vi "Draw Gates On XY Chart.vi"(7 "Micropulse No.":i32, 8 "error in (no error)":errorcluster, 9 "Echo Range":dbl, 10 "XYGraph in":refnum<vi>, 11 "Test No.":u32) -> (0 "error out":errorcluster)   [LabVIEW 2026, in "MicroPulse_Driver.lvlib"]
uses:
  <instrlib>/MicroPulse/MicroPulse_Driver.lvlib
panel:
  out "Picture out":picture
  in  "Picture in":picture
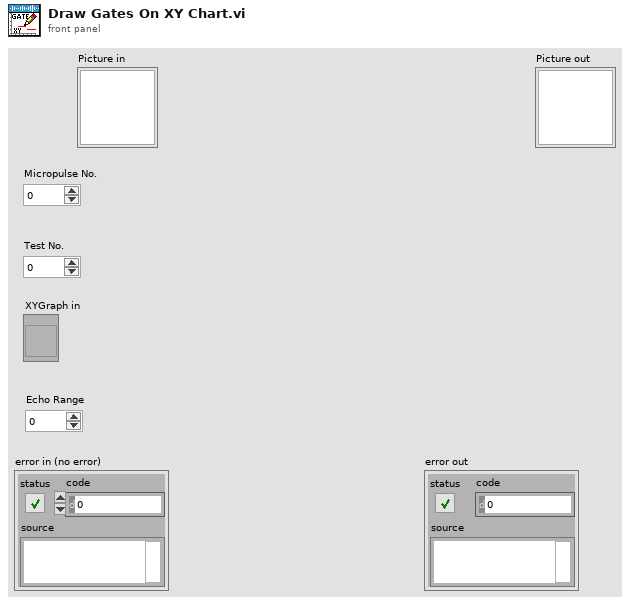
[diagram p1: front panel]
types:
  T1 = cluster{"Start (us)":dbl, "Length (us)":dbl, "Threshold":u16, "Name":string, "Enabled?":bool, "Colour":u32}
  T2 = cluster{"Lable":string, "Visible":bool, "Width":u16, "Colour":u32, "Line":enum32{"Solid", "Dash", "Dot", "DashDot", "DashDotDot"}}
  T3 = typedef "MicroPulse_Driver.lvlib/MP - Registry Gates.ctl" = cluster{"Display Gate":T4, "ETM Mode":T5, "Echo Gate":T6, "Insp Gates":T7[]}
  T4 = typedef "MicroPulse_Driver.lvlib/MP - display gate.ctl" = cluster{"Start":dbl, "Length":dbl}
  T5 = typedef "MicroPulse_Driver.lvlib/MP - echo gate mode.ctl" = enum16{"Echo Trigger OFF", "Echo Gate Display Mode", "Echo Trigger ON", "Multi Gate or FMC Mode", "Reserved", "PA - Echo Trigger ON"}
  T6 = typedef "MicroPulse_Driver.lvlib/MP - echo gate parameters.ctl" = cluster{"Start (us)":dbl, "Length (us)":dbl, "Threshold":u16, "Colour":u32}
  T7 = typedef "MicroPulse_Driver.lvlib/MP - multigate inspection gate parameters.ctl" = cluster{"Start (us)":dbl, "Length (us)":dbl, "Threshold":u16, "Enabled?":bool, "Max # Peaks":u16, "Hysteresis":T8, "Mode":T9, "Inverted?":bool, "Colour ":u32}
  T8 = typedef "MicroPulse_Driver.lvlib/MP - hysteresis level.ctl" = enum16{"None", "3dB", "6dB", "9dB", "12dB"}
  T9 = typedef "MicroPulse_Driver.lvlib/MP - multigate mode.ctl" = enum16{"1st Peak in Gate", "Largest Peak In Gate", "All Peaks In Gate", "1st Threshold Crossing"}
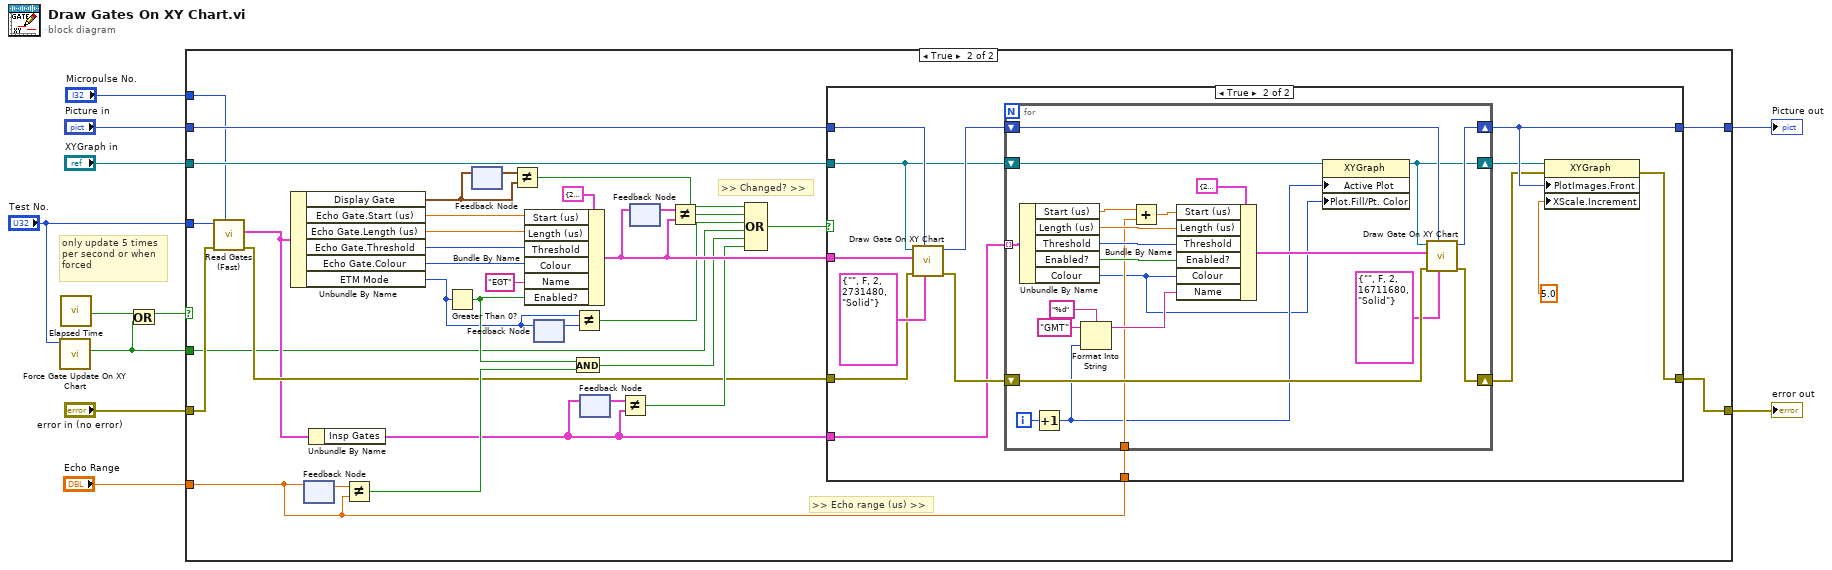
[diagram p0: block diagram]
diagram:
  # "only update 5 times\nper second or when\nforced"
  n1 = call <instrlib>:"Force Gate Update On XY Chart.vi"("Test No."="Test No.") -> ("Update gate display?"=w1:bool)  [unwired: 8 in, 2 out]
  n2 = call "Elapsed Time"() -> ("Time has Elapsed"=w4:bool)  [unwired: 12 in, 7 out]
  n3 = Or(x=w4, y=w1) -> (x .or. y?=w3:bool)
  n4 = case shown="True" w3 {
    tunnel: [w13 w47] -> w11
    tunnel: [w12 w46] -> w10
    tunnel: "Picture in" -> [w13 w45]
    tunnel: "XYGraph in" -> [_ w44]
    tunnel: "Test No." -> [_ w20]
    tunnel: "error in (no error)" -> [w12 w32]
    tunnel: "Micropulse No." -> [_ w30]
    tunnel: "Echo Range" -> [_ w15]
    tunnel: w1 -> [_ w14]
    frame False {
    }
    frame True {
      # ">> Echo range (us) >>"
      # ">> Changed? >>"
      n5 = call <instrlib>:"Read Gates (Fast).vi"("Micropulse # In"=w30, "error in (no error)"=w32, "Test No."=w20) -> ("error out"=w31:errorcluster, "Gates"=w29:T3)  [unwired: 5 in, 2 out]
      n6 = Unbundle By Name(w29) -> ("Display Gate"=w26:T4, "Echo Gate.Start (us)"=w43:dbl, "Echo Gate.Length (us)"=w42:dbl, "Echo Gate.Threshold"=w41:u16, "Echo Gate.Colour"=w16:u32, "ETM Mode"=w17:T5)
      n7 = feedback #1() -> (w35:dbl)  [unwired: 1 in]
      n8 = feedback-in #1(w15) -> ()
      n9 = Unbundle By Name(w29) -> ("Insp Gates"=w28:T7[])
      n10 = Not Equal?(x=w35, y=w15) -> (x != y?=w34:bool)
      n11 = Greater Than 0?(x=w17) -> (x > 0?=w18:bool)
      n12 = feedback #2() -> (w27:T4)  [unwired: 1 in]
      n13 = feedback-in #2(w26) -> ()
      n14 = Not Equal?(x=w27, y=w26) -> (x != y?=w25:bool)
      n15 = Bundle By Name(cluster=T1 {"Start (us)"=2.0, "Length (us)"=7.0, "Threshold"=100, "Name"="", "Enabled?"=FALSE, "Colour"=0} ("Inspection Gate"), "Start (us)"=w43, "Length (us)"=w42, "Threshold"=w41, "Colour"=w16, "Name"="EGT", "Enabled?"=w18) -> (w38:T1)
      n16 = feedback #3() -> (w23:T5)  [unwired: 1 in]
      n17 = feedback-in #3(w17) -> ()
      n18 = And(x=w18, y=w34) -> (x .and. y?=w24:bool)
      n19 = Not Equal?(x=w17, y=w23) -> (x != y?=w21:bool)
      n20 = feedback #4() -> (w37:T7[])  [unwired: 1 in]
      n21 = feedback-in #4(w28) -> ()
      n22 = Not Equal?(x=w37, y=w28) -> (x != y?=w33:bool)
      n23 = feedback #5() -> (w39:T1)  [unwired: 1 in]
      n24 = feedback-in #5(w38) -> ()
      n25 = Not Equal?(x=w39, y=w38) -> (x != y?=w36:bool)
      n26 = Compound Arithmetic op=OR(w25, w36, w21, w14, w24, w33) -> (w22:bool)
      n27 = case shown="True" w22 {
        tunnel: [w48 w63] -> w47
        tunnel: [w49 w60] -> w46
        tunnel: w45 -> [w48 w58]
        tunnel: w31 -> [w49 w56]
        tunnel: w38 -> [_ w51]
        tunnel: w28 -> [_ w52]
        tunnel: w44 -> [_ w54]
        tunnel: w15 -> [_ w53]
        frame False {
        }
        frame True {
          n28 = call <instrlib>:"Draw Gate On XY Chart.vi"("pen"=T2 {"Lable"="", "Visible"=FALSE, "Width"=2, "Colour"=2731480, "Line"=enum."Solid"}, "Picture in"=w58, "error in (no error)"=w56, "Inspection Gate"=w51, "XY Graph"=w54) -> ("error out"=w55:errorcluster, "Picture out"=w57:picture)  [unwired: 5 in]
          n29 = for {
            shift-right: [w84] -> w61
            shift-left: w55 -> [w85]
            shift-right: [w82] -> w63
            shift-left: w57 -> [w83]
            tunnel: w52 -> [w81] mode=indexing
            shift-right: [w66] -> w62
            shift-left: w54 -> [w71]
            tunnel: w53 -> [w68]
            i -> [w73]
            n30 = Unbundle By Name(w81) -> ("Start (us)"=w80:dbl, "Length (us)"=w79:dbl, "Threshold"=w78:u16, "Enabled?"=w76:bool, "Colour"=w64:u32)
            n31 = Increment(x=w73) -> (x+1=w65:i32)
            n32 = Format Into String(format string="%d", initial string="GMT", w65) -> (resulting string=w72:string)  [unwired: 1 in, 1 out]
            n33 = Add(x=w80, y=w68) -> (x+y=w69:dbl)
            n34 = Bundle By Name(cluster=T1 {"Start (us)"=2.0, "Length (us)"=7.0, "Threshold"=100, "Name"="", "Enabled?"=FALSE, "Colour"=0} ("Inspection Gate"), "Start (us)"=w69, "Length (us)"=w79, "Threshold"=w78, "Enabled?"=w76, "Colour"=w64, "Name"=w72) -> (w77:T1)
            n35 = property class="XYGraph"(reference=w71, "Active Plot"=w65, "Plot.Fill/Pt. Color"=w64) -> (reference out=w66:refnum<vi>)  [unwired: 1 in, 1 out]
            n36 = call <instrlib>:"Draw Gate On XY Chart.vi"("pen"=T2 {"Lable"="", "Visible"=FALSE, "Width"=2, "Colour"=16711680, "Line"=enum."Solid"}, "Picture in"=w83, "error in (no error)"=w85, "Inspection Gate"=w77, "XY Graph"=w66) -> ("error out"=w84:errorcluster, "Picture out"=w82:picture)  [unwired: 5 in]
          }
          n37 = property on="Property Node" class="XYGraph"(reference=w62, error in=w61, "PlotImages.Front"=w63, "XScale.Increment"=5.0 ("X Scale.Range:Increment")) -> (error out=w60:errorcluster)  [unwired: 1 out]
        }
      }
    }
  }
  "error out" <- w10
  "Picture out" <- w11
